vi "CAN Frame to Signal.vi"(8 "error in (no error)":errorcluster, 10 "Frame":string, 11 "ENET in":refnum<class "ENET_BS120x.lvclass">) -> (0 "error out":errorcluster, 2 "signal data":dbl[](array[numeric]), 3 "ENET out":refnum<class "ENET_BS120x.lvclass">)   [LabVIEW 2021, in "BS120x Driver.lvlib" / "ENET_BS120x.lvclass"]
uses:
  ENET_BS120x.lvclass
  ENET_BS120x.lvclass/ENET_BS120x.ctl
  _Private/Data Classes/CAN Data Class/CAN Data.lvclass/CAN Data.ctl
  <vilib>/xnet/xnet.llb/XNET Frame CAN.ctl
  <vilib>/xnet/xnet.llb/XNET Frame Type CAN.ctl
  _Private/Data Classes/CAN Data Class/Read CAN Lookup.vi
  <vilib>/xnet/xnet.llb/XNET Create Session (Conversion).vi
  <vilib>/xnet/xnet.llb/XNET Convert (Frame CAN to Signal).vi
  <resource>/objmgr/xnet.rc
  _Private/Data Classes/CAN Data Class/CAN Data.lvclass
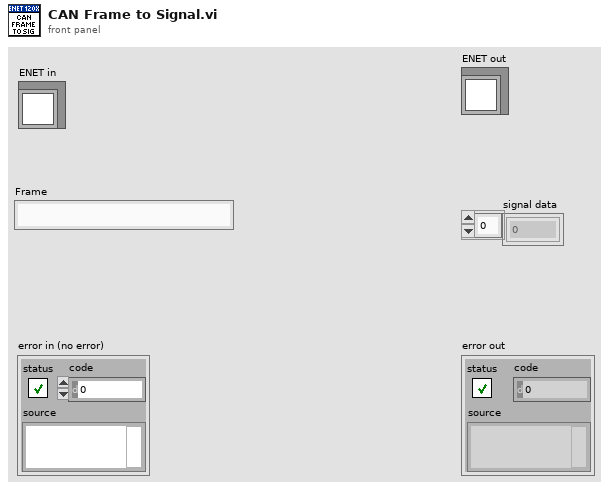
[diagram p1: front panel]
types:
  T1 = typedef "XNET Frame CAN.ctl" = cluster{"timestamp":timestamp, "payload":u8[], "identifier":u32, "type":T2, "extended?":bool, "echo?":bool}
  T2 = typedef "XNET Frame Type CAN.ctl" = u8
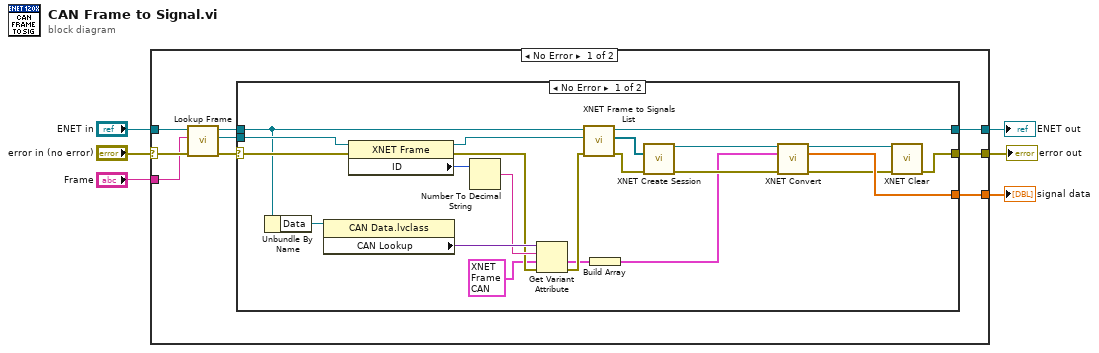
[diagram p0: block diagram]
diagram:
  n1 = case shown="No Error" "error in (no error)" {
    selector: "error in (no error)" -> [w13 w41]
    tunnel: [w12 w41] -> w5
    tunnel: [w9 w40] -> w1
    tunnel: "ENET in" -> [w10 w40]
    tunnel: "Frame" -> [w8 _]
    tunnel: [w11 _] -> w3
    frame No Error {
      n2 = call "Lookup Frame.vi"("error in (no error)"=w13, "Frame"=w8, "Ethernet in"=w10) -> ("error out"=w15:errorcluster, "XNET Frame"=w14:refnum<k21>, "Ethernet out"=w7:refnum<class "ENET_BS120x.lvclass">)  [unwired: 6 in]
      n3 = case shown="No Error" w15 {
        selector: w15 -> [w34 w38]
        tunnel: [w30 w38] -> w12
        tunnel: w14 -> [w37 _]
        tunnel: [w33 _] -> w11
        tunnel: w7 -> [w17 w39]
        tunnel: [w18 w39] -> w9
        frame No Error {
          # "CAN frame found"
          n4 = Unbundle By Name(w17) -> ("Data"=w16:refnum<class "CAN Data.lvclass">)
          n5 = property class="CAN Data.lvclass"(reference=w16) -> ("CAN Lookup"=w28:variant)  [unwired: 1 in, 2 out]
          n6 = property class="XNET Frame"(reference=w37, error in=w34) -> (reference out=w20:refnum<k21>, error out=w25:errorcluster, "ID"=w27:u32)
          n7 = Number To Decimal String(number=w27) -> (decimal integer string=w26:string)  [unwired: 1 in]
          n8 = Get Variant Attribute(Variant=w28, name=w26, default value (empty Variant)=T1 {"timestamp"=timestamp(0 s since 1904-01-01), "payload"=[], "identifier"=0, "type"=0, "extended?"=FALSE, "echo?"=FALSE} ("CAN frame"), error in=w25) -> (value=w23:T1, error out=w24:errorcluster)  [unwired: 2 out]
          n9 = call-dynamic "XNET Frame to Signals List.vi"("error in (no error)"=w24, "XNET Frame"=w20, "BS1200 in"=w17) -> ("error out"=w29:errorcluster, "Sorted XNET Signals"=w19:refnum<k21>[], "BS1200 out"=w18:refnum<class "ENET_BS120x.lvclass">)  [unwired: 6 in]
          n10 = Build Array(w23) -> (w22:T1[])
          n11 = call-poly <vilib>:"XNET Create Session.vi"("signal list"=w19, "error in (no error)"=w29) -> ("session out"=w36:refnum<k21>, "error out"=w35:errorcluster)  [unwired: 12 out]
          n12 = call-poly <vilib>:"XNET Convert.vi"("session in"=w36, "frame data"=w22, "error in (no error)"=w35) -> ("session out"=w32:refnum<k21>, "signal data"=w33:dbl[], "error out"=w31:errorcluster)  [unwired: 10 out]
          n13 = call <vilib>:"XNET Clear.vi"("session in"=w32, "error in (no error)"=w31) -> ("error out"=w30:errorcluster)  [unwired: 13 in]
        }
        frame Error {
        }
      }
    }
    frame Error {
    }
  }
  "error out" <- w5
  "signal data" <- w3
  "ENET out" <- w1
